vi "getColor.vi"(8 "error in (no error)":errorcluster, 10 "Color":string, 11 "ColorFactory in":refnum<class "ColorFactory.lvclass">) -> (0 "error out":errorcluster, 2 "afColor.lvclass":refnum<class "afColor.lvclass">, 3 "ColorFactory out":refnum<class "ColorFactory.lvclass">)   [LabVIEW 2017, in "ColorFactory.lvclass"]
uses:
  ColorFactory.lvclass
  afColor Class/afColor.lvclass
  afRed Class/afRed.lvclass
  C:/Users/fflores/Documents/LabVIEW-Open-Projects/LabIVEW OOP Design Patterns/Abstract Factory Pattern/afColor Class/afColor.lvclass
  afBlue Class/afBlue.lvclass
  afGreen Class/afGreen.lvclass
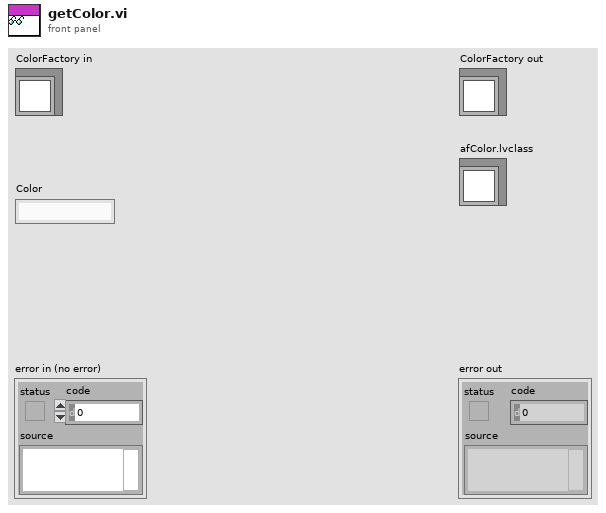
[diagram p1: front panel]
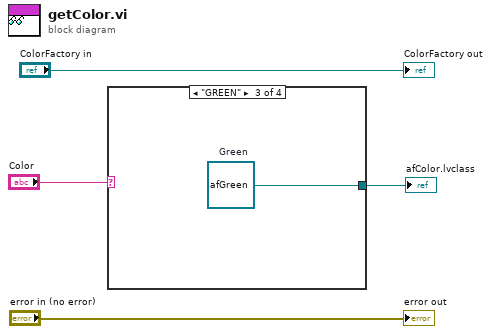
[diagram p0: block diagram]
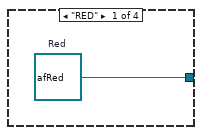
[diagram p2: hidden frame]
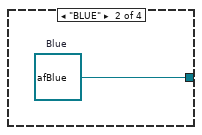
[diagram p3: hidden frame]
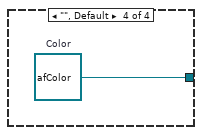
[diagram p4: hidden frame]
diagram:
  n1 = case shown="\"GREEN\"" "Color" {
    tunnel: [w5 w6 w7 w8] -> w1
    frame "RED" {
      w5 = refnum<class "afRed.lvclass"> refnum  # Red
    }
    frame "BLUE" {
      w6 = refnum<class "afBlue.lvclass"> refnum  # Blue
    }
    frame "GREEN" {
      w7 = refnum<class "afGreen.lvclass"> refnum  # Green
    }
    frame "", Default {
      w8 = refnum<class "afColor.lvclass"> refnum  # Color
    }
  }
  "afColor.lvclass" <- w1
  "error out" <- "error in (no error)"
  "ColorFactory out" <- "ColorFactory in"
